vi "unique-name-multiple-instances.vi"(8 "error in (no error)":errorcluster) -> (0 "error out":errorcluster)   [LabVIEW 2013]
uses:
  src/SMO/SMO.lvclass
  <vilib>/addons/_JKI Toolkits/Caraya/classes/Test/Test.lvclass
  <vilib>/addons/_JKI Toolkits/Caraya/classes/Assert/Assert.lvclass
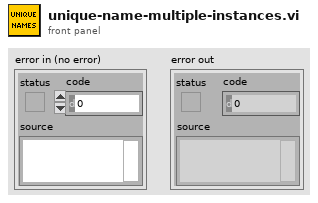
[diagram p1: front panel]
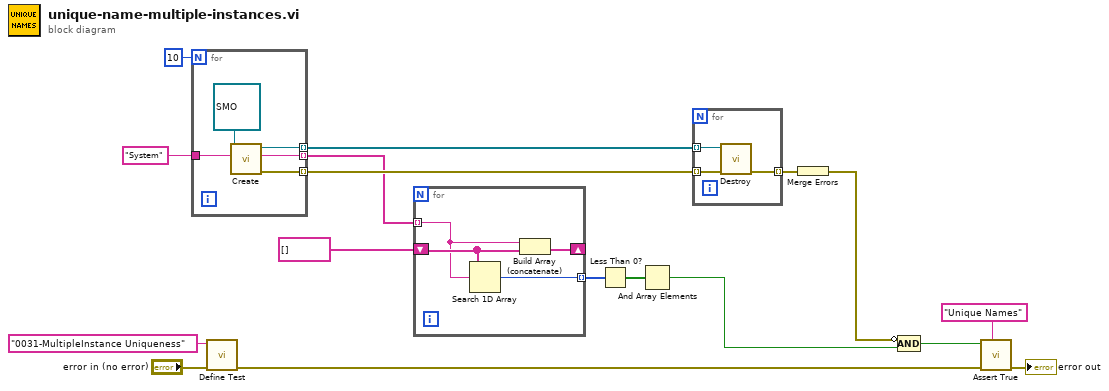
[diagram p0: block diagram]
diagram:
  n1 = for {
    N: 10 -> [_]
    tunnel: "System" ("Subsystem Name (optional)") -> [w21]
    tunnel: [w20] -> w4 mode=indexing
    tunnel: [w19] -> w10 mode=indexing
    tunnel: [w18] -> w7 mode=indexing
    n2 = call "Create.vi"("Subsystem Name (optional)"=w21, "SMO"=refnum<class "SMO.lvclass"> refnum ("SMO.lvclass")) -> ("error out"=w18:errorcluster, "SMO name"=w20:string, "SMO out"=w19:refnum<class "SMO.lvclass">)  [unwired: 7 in]
  }
  n3 = call <vilib>:"Define Test.vi"("error in (no error)"="error in (no error)", "Label (VI Title)"="0031-MultipleInstance Uniqueness") -> ("error out"=w6:errorcluster)  [unwired: 9 in]
  n4 = for {
    shift-right: [w24] -> _
    shift-left: string[] [] -> [w26]
    tunnel: w4 -> [w25] mode=indexing
    tunnel: [w23] -> w3 mode=indexing
    n5 = Search 1D Array(1D array=w26, element=w25) -> (index of element=w23:i32)  [unwired: 1 in]
    n6 = Build Array (concatenate)(w25, w26) -> (w24:string[])
  }
  n7 = Less Than 0?(x=w3) -> (x < 0?=w2:bool[])
  n8 = And Array Elements(Boolean array=w2) -> (logical AND=w1:bool)
  n9 = for {
    tunnel: w10 -> [w29] mode=indexing
    tunnel: [w28] -> w9 mode=indexing
    tunnel: w7 -> [w27] mode=indexing
    n10 = call "Destroy.vi"("error in (no error)"=w27, "SMO"=w29) -> ("error out"=w28:errorcluster)  [unwired: 9 in]
  }
  n11 = Merge Errors(w9) -> (w8:errorcluster)
  n12 = Compound Arithmetic op=AND(invert w8, w1) -> (w13:bool)
  n13 = call <vilib>:"Assert True.vi"("Label"="Unique Names" ("Label (VI Title)"), "error in (no error)"=w6, "True?"=w13) -> ("error out"=→"error out":errorcluster)  [unwired: 8 in]
